vi "Read ColHeaders.vi"(8 "error in (no error)":errorcluster, 11 "CarexMData in":refnum<class "ExpData.lvclass">) -> (0 "error out":errorcluster, 2 "ColHeaders":cluster{"Name":string, "Index":i8, "Size":i8}[](array[cluster]), 3 "CarexMData out":refnum<class "ExpData.lvclass">)   [LabVIEW 2016, in "ExpData.lvclass"]
uses:
  ExpData.lvclass
  ExpData.lvclass/ExpData.ctl
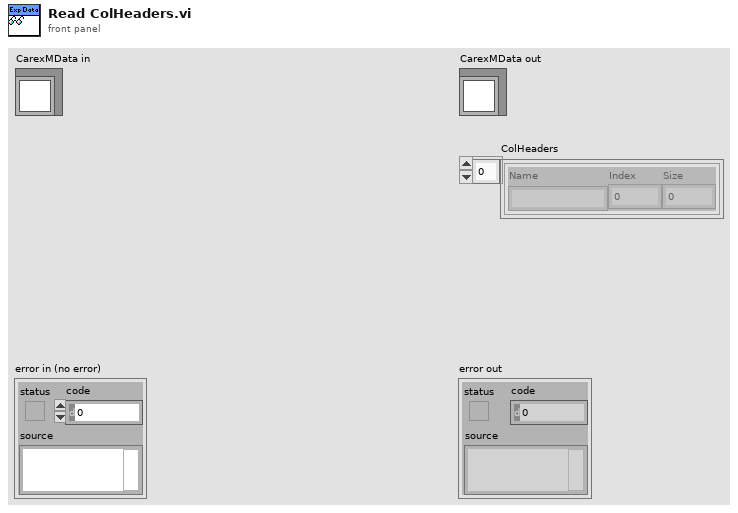
[diagram p1: front panel]
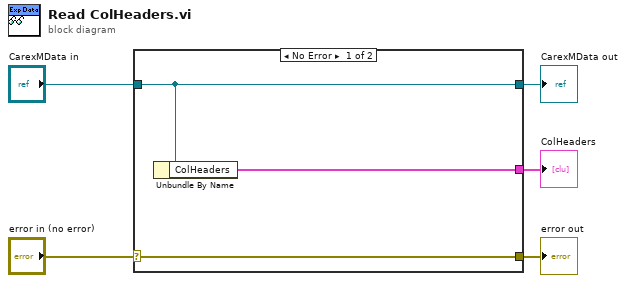
[diagram p0: block diagram]
diagram:
  n1 = case shown="No Error" "error in (no error)" {
    selector: "error in (no error)" -> [w8 w9]
    tunnel: [w8 w9] -> w4
    tunnel: [w7 w10] -> w2
    tunnel: "CarexMData in" -> [w7 w10]
    tunnel: [w6 _] -> w1
    frame No Error {
      n2 = Unbundle By Name(w7) -> ("ColHeaders"=w6:cluster{"Name":string, "Index":i8, "Size":i8}[])
    }
    frame Error {
    }
  }
  "error out" <- w4
  "CarexMData out" <- w2
  "ColHeaders" <- w1
